vi "FlatToRichcif_manager_ClockStatus.vi"(5 "OutputClusterType":T1, 11 "InputCluster":T4) -> (3 "OutputCluster":T1)   [LabVIEW 2021, in "CIF_Launcher_client.lvlib"]
uses:
  CIF_Launcher_client.lvlib
  cif_manager_ClockStatus_Flat.ctl
  cif_manager_ClockConversion_Flat.ctl
  cif_manager_TimePair_Flat.ctl
  cif_manager_ClockStatus.ctl
  cif_manager_ClockConversion.ctl
  cif_manager_TimePair.ctl
  FlatToRichcif_manager_TimePair.vi
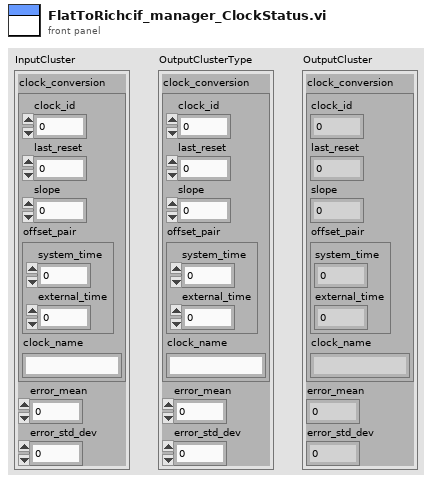
[diagram p1: front panel]
types:
  T1 = typedef "CIF_Launcher_client.lvlib/cif_manager_ClockStatus.ctl" = cluster{"clock_conversion":T2, "error_mean":i64, "error_std_dev":i64}
  T2 = typedef "CIF_Launcher_client.lvlib/cif_manager_ClockConversion.ctl" = cluster{"clock_id":u32, "last_reset":i64, "slope":dbl, "offset_pair":T3, "clock_name":string}
  T3 = typedef "CIF_Launcher_client.lvlib/cif_manager_TimePair.ctl" = cluster{"system_time":i64, "external_time":i64}
  T4 = typedef "CIF_Launcher_client.lvlib/cif_manager_ClockStatus_Flat.ctl" = cluster{"clock_conversion":T5, "error_mean":i64, "error_std_dev":i64}
  T5 = typedef "CIF_Launcher_client.lvlib/cif_manager_ClockConversion_Flat.ctl" = cluster{"clock_id":u32, "last_reset":i64, "slope":dbl, "offset_pair":T6, "clock_name":string}
  T6 = typedef "CIF_Launcher_client.lvlib/cif_manager_TimePair_Flat.ctl" = cluster{"system_time":i64, "external_time":i64}
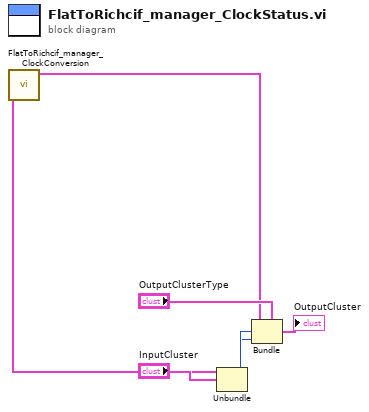
[diagram p0: block diagram]
diagram:
  n1 = Unbundle "Unbundle"("InputCluster") -> ("clock_conversion"=w4:T5, "error_mean"=w2:i64, "error_std_dev"=w1:i64)
  n2 = call "FlatToRichcif_manager_ClockConversion.vi"("InputCluster"=w4) -> ("OutputCluster"=w3:T2)  [unwired: 10 in]
  n3 = Bundle "Bundle"(cluster="OutputClusterType", "clock_conversion"=w3, "error_mean"=w2, "error_std_dev"=w1) -> (→"OutputCluster":T1)
